vi "Test MQTT API.vi"() -> ()   [LabVIEW 2015, in "MQTT.lvlib"]
doc: "MQTT API Tester."
uses:
  MQTT.lvlib
panel:
  in  "Tab Control":enum32{"Config", "Connection", "Sub", "Pub"}(tab)
  in  "conf":bool
  in  "JSON config":string
  in  "disconn":bool
  in  "conn":bool
  in  "unsubscribe":bool
  in  "subscribe":bool
  in  "Topic":string
  in  "Payload":string
  in  "Topic Pub":string
  in  "PUB":bool
  in  "Run as Singleton?":bool
  in  "Show Block Diagram":bool
  in  "Refresh Modules":bool
  out "Active Modules":string[](array[string])
  in  "Stop Module":bool
  in  "Select Module":i32(ring)=-1 caption="Select Module\nTo send Request to" items=["All"=-1]
  in  "Run New Module":bool
  in  "Hide Module Panel":bool
  in  "Show Module Panel":bool
  out "Status":string
  # "This VI tests the API for the Module."
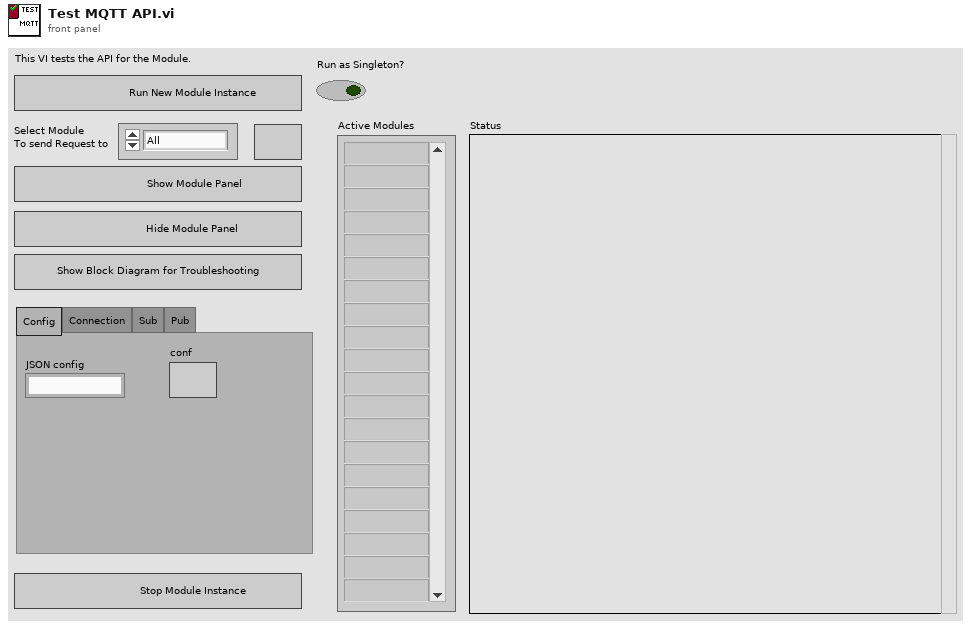
[diagram p1: front panel]
types:
  T1 = typedef "MQTT.lvlib/Broadcast Events--cluster.ctl" = cluster{"Module Did Init":refnum<user-event>, "Status Updated":refnum<user-event>, "Error Reported":refnum<user-event>, "Module Did Stop":refnum<user-event>, "Update Module Execution Status":refnum<user-event>, "Message":refnum<user-event>}
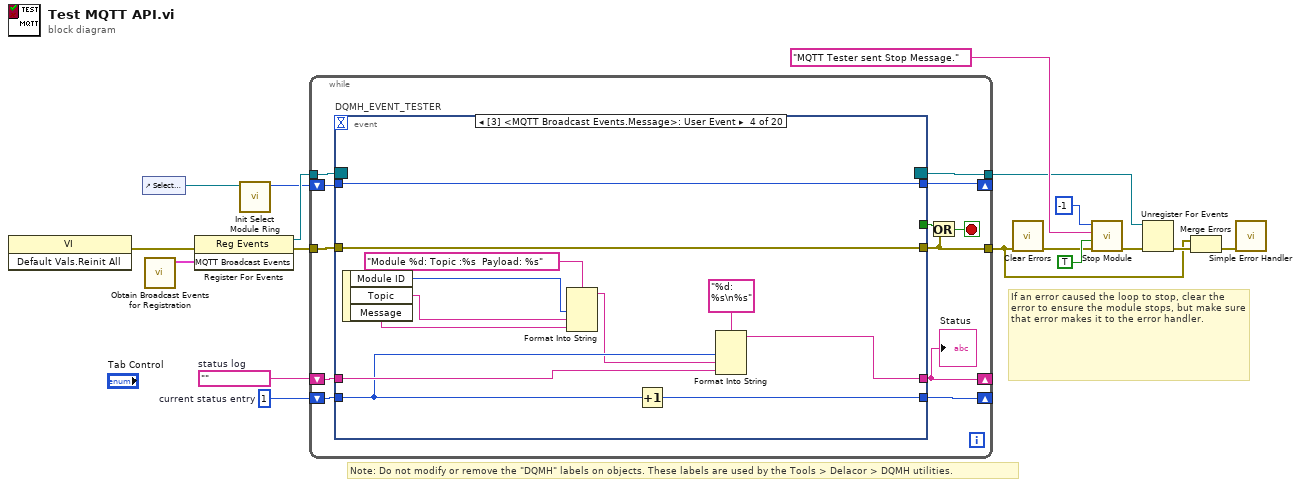
[diagram p0: block diagram]
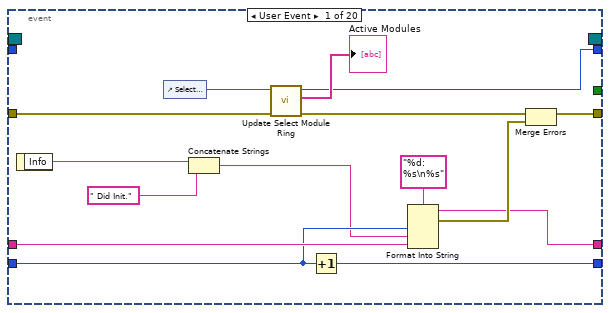
[diagram p2: hidden frame]
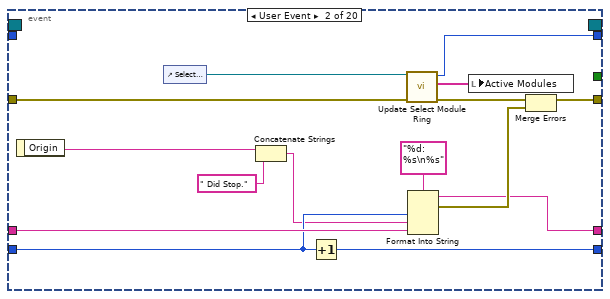
[diagram p3: hidden frame]
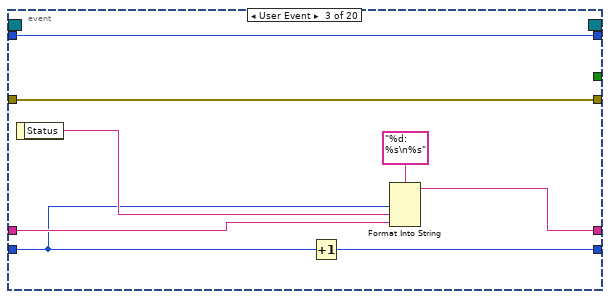
[diagram p4: hidden frame]
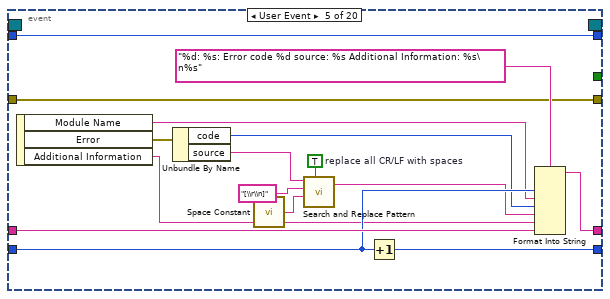
[diagram p5: hidden frame]
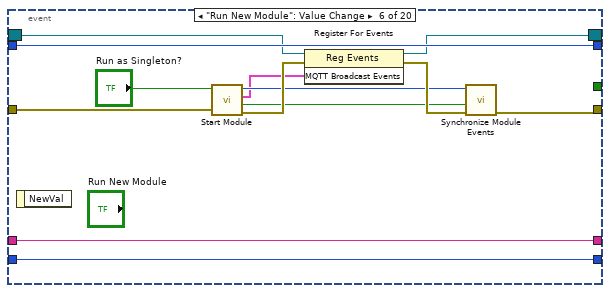
[diagram p6: hidden frame]
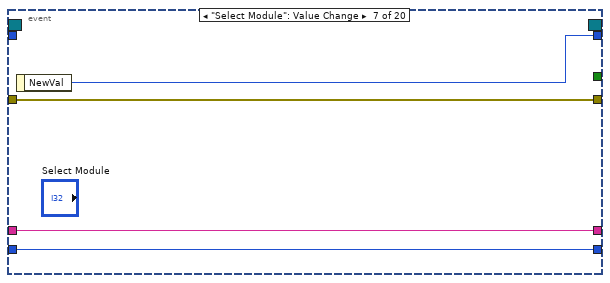
[diagram p7: hidden frame]
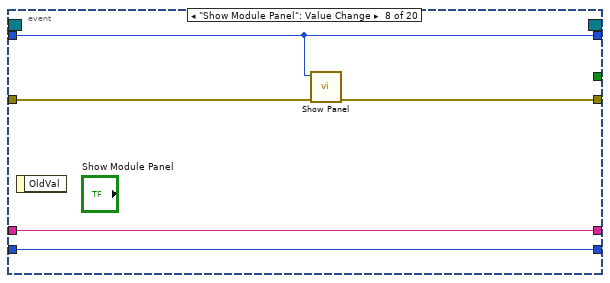
[diagram p8: hidden frame]
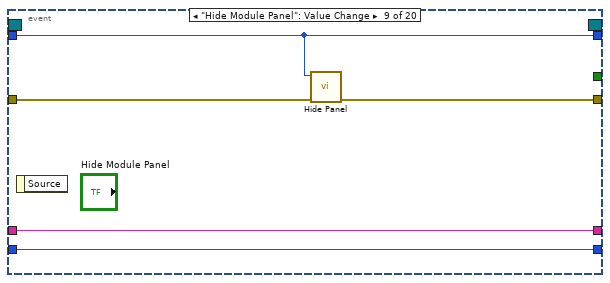
[diagram p9: hidden frame]
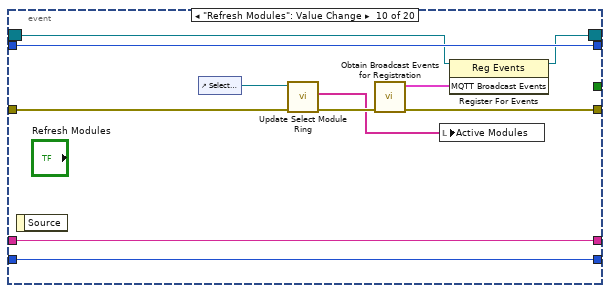
[diagram p10: hidden frame]
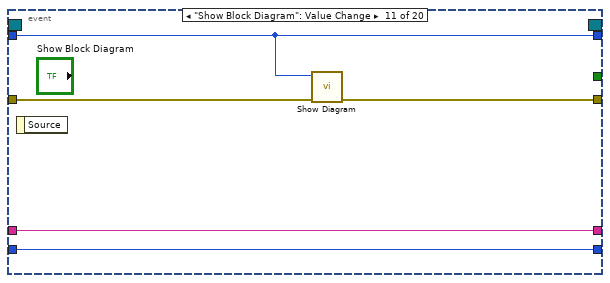
[diagram p11: hidden frame]
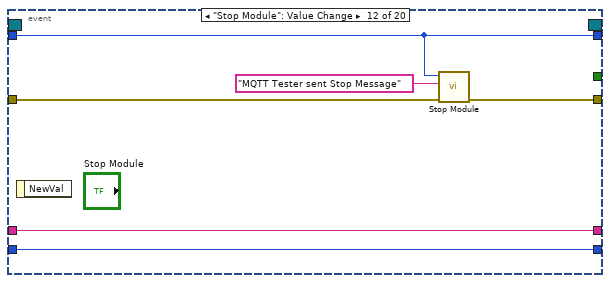
[diagram p12: hidden frame]
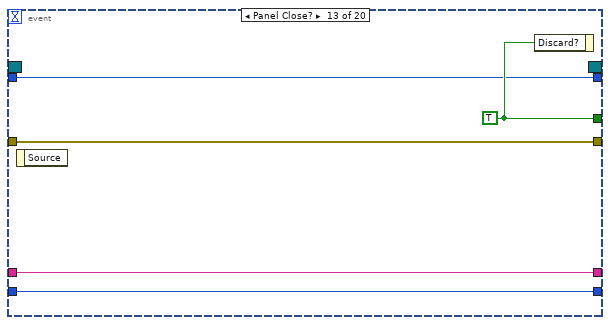
[diagram p13: hidden frame]
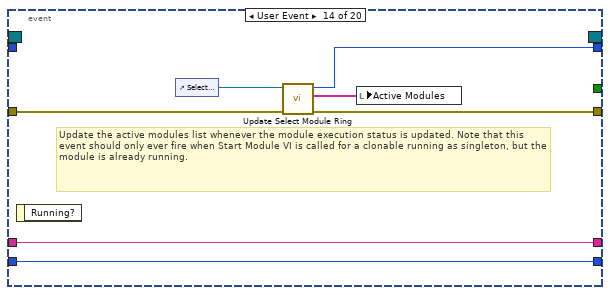
[diagram p14: hidden frame]
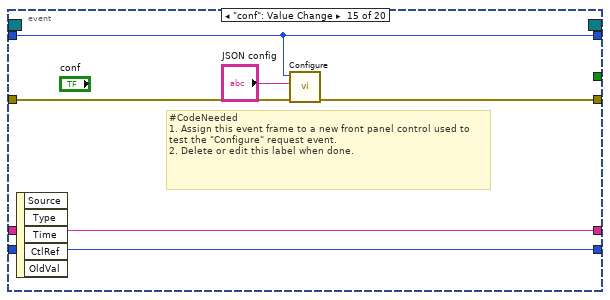
[diagram p15: hidden frame]
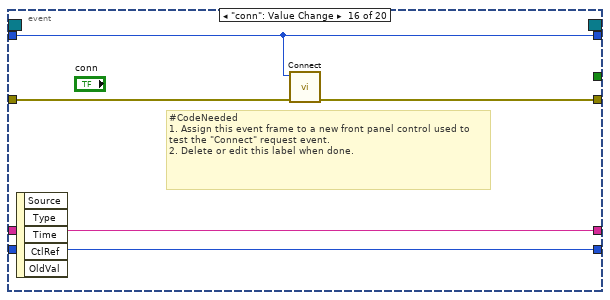
[diagram p16: hidden frame]
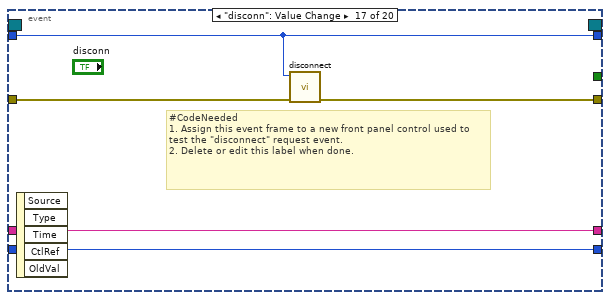
[diagram p17: hidden frame]
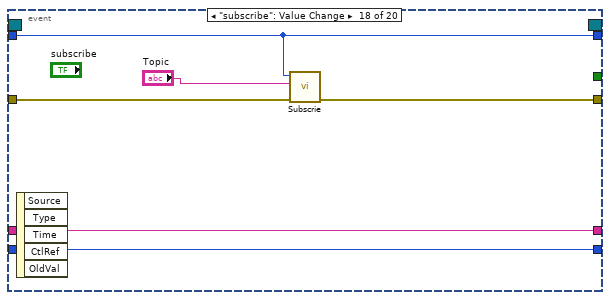
[diagram p18: hidden frame]
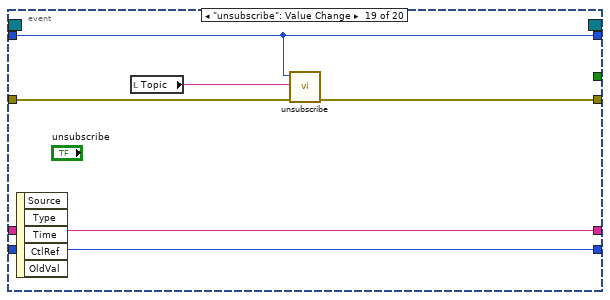
[diagram p19: hidden frame]
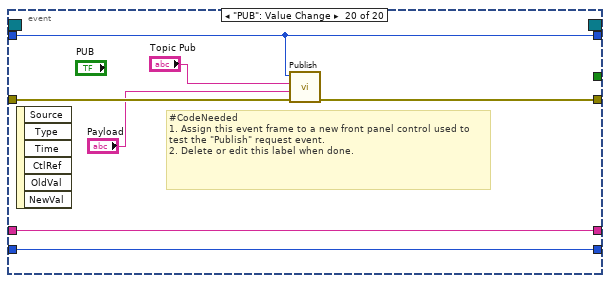
[diagram p20: hidden frame]
diagram:
  w13 = 1  # current status entry
  w14 = ""  # status log
  # "If an error caused the loop to stop, clear the error to ensure the module stops, but make sure that error makes it to the error handler."
  # "Note: Do not modify or remove the \"DQMH\" labels on objects. These labels are used by the Tools > Delacor > DQMH utilities."
  n1 = invoke class="VI" method="Default Vals.Reinit All"() -> (error out=w6:errorcluster)  [unwired: 3 in, 2 out]
  n2 = control-ref of="Select Module"() -> (w11:refnum<vi>)
  n3 = call "Obtain Broadcast Events for Registration.vi"() -> ("MQTT Broadcast Events"=w10:T1)  [unwired: 10 in, 1 out]
  n4 = register-events(error in=w6, w10) -> (reference out=w17:refnum<event-registration>, error out=w9:errorcluster)  [unwired: 1 in]
  n5 = call "Init Select Module Ring.vi"("Select Module Ring Ref"=w11) -> ("Value for All Modules"=w12:i32)  [unwired: 8 in, 2 out]
  n6 = while {
    tunnel: w17 -> [w29]
    tunnel: [w18] -> w1
    tunnel: w9 -> [w27]
    shift-right: [w23] -> _
    shift-left: w14 -> [w25]
    shift-right: [w24] -> _
    shift-left: w13 -> [w26]
    shift-right: [w20] -> _
    shift-left: w12 -> [w21]
    tunnel: [w19] -> w5
    stop <- w22 stop-if-true
    n7 = event "DQMH_EVENT_TESTER" shown="[3] <MQTT Broadcast Events.Message>: User Event" {
      selector: w29 -> [_ _ _ _ _ w102 _ _ _ w128 _ _ _ _ _ _ _ _ _ _]
      dyn-events: [_ _ _ _ _ w101 _ _ _ w127 _ _ _ _ _ _ _ _ _ _] -> w19
      timeout: _ -> [_ _ _ _ _ _ _ _ _ _ _ _ _ _ _ _ _ _ _ _]
      tunnel: [_ _ _ _ _ _ _ _ _ _ _ _ w149 _ _ _ _ _ _ _] -> w28
      tunnel: [w33 w51 w67 w79 w85 w100 w112 w116 w121 w124 w135 w140 w148 w152 w159 w164 w169 w175 w181 w188] -> w18
      tunnel: w27 -> [w35 w53 w67 w79 w85 w103 w112 w117 w122 w129 w138 w141 w148 w153 w162 w167 w172 w178 w184 w191]
      tunnel: w26 -> [w41 w56 w60 w73 w91 w105 w110 w114 w119 w132 w136 w143 w146 w155 w160 w165 w170 w176 w182 w189]
      tunnel: w25 -> [w42 w57 w63 w75 w93 w106 w111 w115 w120 w133 w137 w144 w147 w156 w161 w166 w171 w177 w183 w190]
      tunnel: [w39 w54 w64 w76 w88 w106 w111 w115 w120 w133 w137 w144 w147 w156 w161 w166 w171 w177 w183 w190] -> w23
      tunnel: [w40 w55 w66 w78 w94 w105 w110 w114 w119 w132 w136 w143 w146 w155 w160 w165 w170 w176 w182 w189] -> w24
      tunnel: w21 -> [_ _ w61 w74 w95 w104 _ w113 w118 w131 w134 w142 w145 _ w158 w163 w168 w173 w179 w187]
      tunnel: [w30 w48 w61 w74 w95 w104 w109 w113 w118 w131 w134 w142 w145 w151 w158 w163 w168 w173 w179 w187] -> w20
      event User Event {
        n8 = event-data() -> ("Info"=w38:string)  [unwired: 1 in]
        n9 = control-ref of="Select Module"() -> (w32:refnum<vi>)
        n10 = Concatenate Strings(w38, " Did Init.") -> (w37:string)
        n11 = call "Update Select Module Ring.vi"("error in (no error)"=w35, "Select Module Ring Ref"=w32) -> ("error out"=w34:errorcluster, "Active Modules (Array)"=→"Active Modules":string[], "New Module Ring Value"=w30:i32)  [unwired: 7 in]
        n12 = Increment(x=w41) -> (x+1=w40:i32)
        n13 = Format Into String(format string="%d: %s\n%s", w41, w37, w42) -> (resulting string=w39:string, error out=w44:errorcluster)  [unwired: 2 in]
        n14 = Merge Errors(w34, w44) -> (w33:errorcluster)
      }
      event User Event {
        n15 = event-data() -> ("Origin"=w46:string)  [unwired: 1 in]
        n16 = control-ref of="Select Module"() -> (w50:refnum<vi>)
        n17 = Concatenate Strings(w46, " Did Stop.") -> (w45:string)
        n18 = Increment(x=w56) -> (x+1=w55:i32)
        n19 = call "Update Select Module Ring.vi"("error in (no error)"=w53, "Select Module Ring Ref"=w50) -> ("error out"=w52:errorcluster, "Active Modules (Array)"=w49:string[], "New Module Ring Value"=w48:i32)  [unwired: 7 in]
        n20 = Format Into String(format string="%d: %s\n%s", w56, w45, w57) -> (resulting string=w54:string, error out=w59:errorcluster)  [unwired: 2 in]
        n21 = local write "Active Modules"(w49) -> ()
        n22 = Merge Errors(w52, w59) -> (w51:errorcluster)
      }
      event User Event {
        n23 = event-data() -> ("Status"=w62:string)  [unwired: 1 in]
        n24 = Increment(x=w60) -> (x+1=w66:i32)
        n25 = Format Into String(format string="%d: %s\n%s", w60, w62, w63) -> (resulting string=w64:string)  [unwired: 2 in, 1 out]
      }
      event User Event {
        n26 = event-data() -> ("Module ID"=w72:i32, "Topic"=w71:string, "Message"=w70:string)  [unwired: 1 in]
        n27 = Format Into String(format string="Module %d: Topic :%s  Payload: %s", w72, w71, w70) -> (resulting string=w69:string)  [unwired: 2 in, 1 out]
        n28 = Increment(x=w73) -> (x+1=w78:i32)
        n29 = Format Into String(format string="%d: %s\n%s", w73, w69, w75) -> (resulting string=w76:string)  [unwired: 2 in, 1 out]
      }
      event User Event {
        w89 = TRUE  # replace all CR/LF with spaces
        n30 = event-data() -> ("Module Name"=w83:string, "Error"=w82:errorcluster, "Additional Information"=w80:string)  [unwired: 1 in]
        n31 = Unbundle By Name(w82) -> ("code"=w84:i32, "source"=w86:string)
        n32 = call <vilib>:"Space Constant.vi"() -> ("String"=w90:string)
        n33 = call <vilib>:"Search and Replace Pattern.vi"("string"=w86, "regular expression (\"\")"="[\\r\\n]" ("regular expression (\"\")"), "replace string (\"\")"=w90, "replace all? (F)"=w89) -> ("result string"=w87:string)  [unwired: 1 in, 1 out]
        n34 = Increment(x=w91) -> (x+1=w94:i32)
        n35 = Format Into String(format string="%d: %s: Error code %d source: %s Additional Information: %s\n%s", w91, w83, w84, w87, w80, w93) -> (resulting string=w88:string)  [unwired: 2 in, 1 out]
      }
      event "Run New Module": Value Change {
        n36 = event-data() -> ()  [unwired: 1 in, 1 out]
        n37 = call "Start Module.vi"("error in (no error)"=w103, "Run as Singleton? (F)"="Run as Singleton?") -> ("error out"=w107:errorcluster, "Wait for Event Sync?"=w98:bool, "MQTT Broadcast Events"=w97:T1, "Module ID"=w99:i32)  [unwired: 6 in]
        n38 = register-events(reference=w102, error in=w107, w97) -> (reference out=w101:refnum<event-registration>, error out=w108:errorcluster)
        n39 = call "Synchronize Module Events.vi"("error in (no error)"=w108, "Wait for Event Sync?"=w98, "Module ID"=w99) -> ("error out"=w100:errorcluster)  [unwired: 7 in, 1 out]
      }
      event "Select Module": Value Change {
        n40 = event-data() -> ("NewVal"=w109:i32)  [unwired: 1 in]
      }
      event "Show Module Panel": Value Change {
        n41 = event-data() -> ()  [unwired: 1 in, 1 out]
        n42 = call "Show Panel.vi"("error in (no error)"=w117, "Module ID"=w113) -> ("error out"=w116:errorcluster)  [unwired: 9 in]
      }
      event "Hide Module Panel": Value Change {
        n43 = event-data() -> ()  [unwired: 1 in, 1 out]
        n44 = call "Hide Panel.vi"("error in (no error)"=w122, "Module ID"=w118) -> ("error out"=w121:errorcluster)  [unwired: 9 in]
      }
      event "Refresh Modules": Value Change {
        n45 = event-data() -> ()  [unwired: 1 in, 1 out]
        n46 = control-ref of="Select Module"() -> (w130:refnum<vi>)
        n47 = call "Update Select Module Ring.vi"("error in (no error)"=w129, "Select Module Ring Ref"=w130) -> ("error out"=w125:errorcluster, "Active Modules (Array)"=w123:string[])  [unwired: 7 in, 1 out]
        n48 = call "Obtain Broadcast Events for Registration.vi"("error in (no error)"=w125) -> ("error out"=w124:errorcluster, "MQTT Broadcast Events"=w126:T1)  [unwired: 9 in]
        n49 = local write "Active Modules"(w123) -> ()
        n50 = register-events(reference=w128, w126) -> (reference out=w127:refnum<event-registration>)  [unwired: 1 in, 1 out]
      }
      event "Show Block Diagram": Value Change {
        n51 = event-data() -> ()  [unwired: 1 in, 1 out]
        n52 = call "Show Diagram.vi"("error in (no error)"=w138, "Module ID"=w134) -> ("error out"=w135:errorcluster)  [unwired: 9 in]
      }
      event "Stop Module": Value Change {
        n53 = event-data() -> ()  [unwired: 1 in, 1 out]
        n54 = call "Stop Module.vi"("error in (no error)"=w141, "Origin"="MQTT Tester sent Stop Message", "Module ID"=w142) -> ("error out"=w140:errorcluster)  [unwired: 8 in]
      }
      event Panel Close? {
        w149 = TRUE ("Discard?")
        n55 = event-data() -> ()  [unwired: 1 in, 1 out]
        n56 = event-data("Discard?"=w149) -> ()  [unwired: 1 in, 1 out]
      }
      event User Event {
        # "Update the active modules list whenever the module execution status is updated. Note that this event should only ever fire when Start Module VI is called for a clonable running as singleton, but the module is already running."
        n57 = event-data() -> ()  [unwired: 1 in, 1 out]
        n58 = control-ref of="Select Module"() -> (w154:refnum<vi>)
        n59 = call "Update Select Module Ring.vi"("error in (no error)"=w153, "Select Module Ring Ref"=w154) -> ("error out"=w152:errorcluster, "Active Modules (Array)"=w150:string[], "New Module Ring Value"=w151:i32)  [unwired: 7 in]
        n60 = local write "Active Modules"(w150) -> ()
      }
      event "conf": Value Change {
        # "#CodeNeeded\n1. Assign this event frame to a new front panel control used to test the \"Configure\" request event.\n2. Delete or edit this label when done."
        n61 = event-data() -> ()  [unwired: 1 in, 5 out]
        n62 = call "Configure.vi"("error in (no error)"=w162, "JSON config"="JSON config", "Module ID"=w158) -> ("error out"=w159:errorcluster)  [unwired: 8 in]
      }
      event "conn": Value Change {
        # "#CodeNeeded\n1. Assign this event frame to a new front panel control used to test the \"Connect\" request event.\n2. Delete or edit this label when done."
        n63 = event-data() -> ()  [unwired: 1 in, 5 out]
        n64 = call "Connect.vi"("error in (no error)"=w167, "Module ID"=w163) -> ("error out"=w164:errorcluster)  [unwired: 9 in]
      }
      event "disconn": Value Change {
        # "#CodeNeeded\n1. Assign this event frame to a new front panel control used to test the \"disconnect\" request event.\n2. Delete or edit this label when done."
        n65 = event-data() -> ()  [unwired: 1 in, 5 out]
        n66 = call "disconnect.vi"("error in (no error)"=w172, "Module ID"=w168) -> ("error out"=w169:errorcluster)  [unwired: 9 in]
      }
      event "subscribe": Value Change {
        n67 = event-data() -> ()  [unwired: 1 in, 5 out]
        n68 = call "Subscrie.vi"("error in (no error)"=w178, "String"="Topic", "Module ID"=w173) -> ("error out"=w175:errorcluster)  [unwired: 8 in]
      }
      event "unsubscribe": Value Change {
        n69 = event-data() -> ()  [unwired: 1 in, 5 out]
        n70 = local read "Topic"() -> (w180:string)
        n71 = call "unsubscribe.vi"("error in (no error)"=w184, "Topic"=w180, "Module ID"=w179) -> ("error out"=w181:errorcluster)  [unwired: 8 in]
      }
      event "PUB": Value Change {
        # "#CodeNeeded\n1. Assign this event frame to a new front panel control used to test the \"Publish\" request event.\n2. Delete or edit this label when done."
        n72 = event-data() -> ()  [unwired: 1 in, 6 out]
        n73 = call "Publish.vi"("error in (no error)"=w191, "Payload"="Payload", "Topic"="Topic Pub", "Module ID"=w187) -> ("error out"=w188:errorcluster)  [unwired: 7 in]
      }
    }
    "Status" <- w23
    n74 = Or(x=w28, y=w18) -> (x .or. y?=w22:bool)
  }
  n75 = call <vilib>:"Clear Errors.vi"("error in (no error)"=w1) -> ("error out"=w3:errorcluster)  [unwired: 5 in, 1 out]
  n76 = call "Stop Module.vi"("error in (no error)"=w3, "Wait for Module to stop? (F)"=TRUE ("Wait for Module to stop?"), "Origin"="MQTT Tester sent Stop Message.", "Module ID"=-1 ("Stop all")) -> ("error out"=w15:errorcluster)  [unwired: 7 in]
  n77 = Unregister For Events(event registration refnum=w5, error in=w15) -> (error out=w16:errorcluster)
  n78 = Merge Errors(w1, w16) -> (w2:errorcluster)
  n79 = call <vilib>:"Simple Error Handler.vi"("error in (no error)"=w2) -> ()  [unwired: 4 in, 5 out]
